vi "readStickEnc.vi"(6 "Reset Counter":bool, 7 "Reverse ENC?":bool, 8 "error in (no error)":errorcluster) -> (0 "error out":errorcluster, 2 "StickEncoder (deg)":dbl)   [LabVIEW 2019, in "SJCube_KNRm.lvlib"]
uses:
  SJCube_KNRm.lvlib
  KNRm_ReMi_OS5.lvlibp/KNRm_ReMi_Toolkit/IO/LowLevel/IO_Channel_Motor.ctl
  KNRm_ReMi_OS5.lvlibp
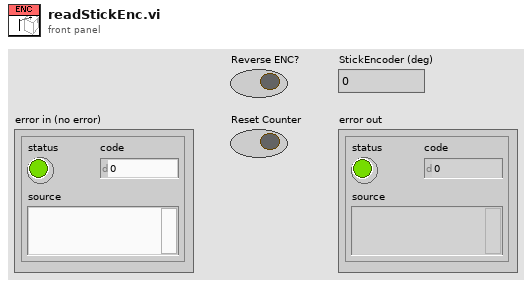
[diagram p1: front panel]
types:
  T1 = typedef "KNRm_ReMi_OS5.lvlibp/IO_Channel_Motor.ctl" = enum16{"M1", "M2", "M3", "M4"}
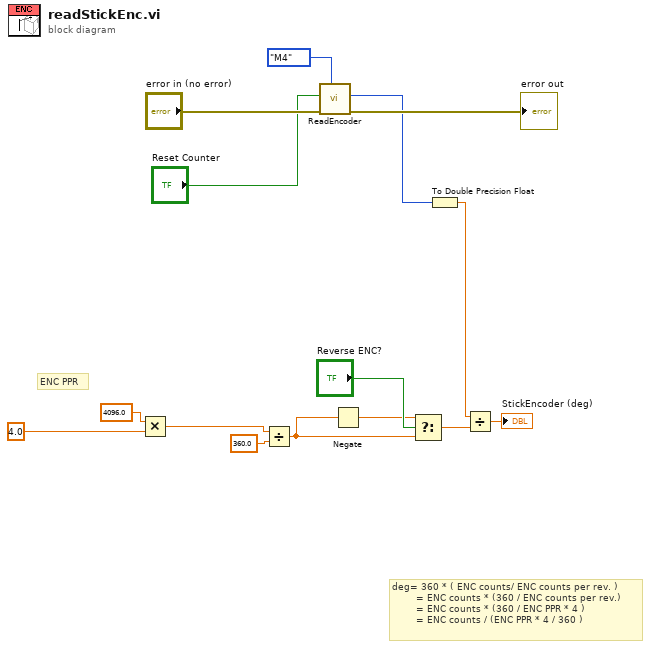
[diagram p0: block diagram]
diagram:
  # "deg= 360 * ( ENC counts/ ENC counts per rev. )\n        = ENC counts * (360 / ENC counts per rev.)\n        = ENC counts * (360 / ENC PPR * 4 )\n        = ENC counts / (ENC PPR * 4 / 360 )"
  # "ENC PPR"
  n1 = Multiply(x=4096.0 ("y"), y=4.0) -> (x*y=w8:dbl)
  n2 = Divide(x=w8, y=360.0) -> (x/y=w6:dbl)
  n3 = call "ReadEncoder.vi"("Channel"=IO_Channel_Motor."M4", "error in"="error in (no error)", "Reset"="Reset Counter") -> ("error out"=→"error out":errorcluster, "ENC (count)"=w1:i32)  [unwired: 7 in]
  n4 = Negate(x=w6) -> (-x=w11:dbl)
  n5 = Select(t=w11, s="Reverse ENC?", f=w6) -> (s? t:f=w12:dbl)
  n6 = To Double Precision Float(number=w1) -> (double precision float=w14:dbl)
  n7 = Divide(x=w14, y=w12) -> (x/y=→"StickEncoder (deg)":dbl)
